vi "test2-DifferentChainNodesProcessDifferentAllowedMessages.vi"(8 "error in (no error)":errorcluster, 11 "TestCase in":refnum<class "testcase-CSMChainMode.lvclass">) -> (0 "error out":errorcluster, 3 "TestCase out":refnum<class "testcase-CSMChainMode.lvclass">)   [LabVIEW 2017, in "testcase-CSMChainMode.lvclass"]
uses:
  testcase-CSMChainMode.lvclass
  <vilib>/addons/_JKI Toolkits/VI Tester/TestCase.llb/TestCase.lvclass
  src/user.lib/_NEVSTOP/Communicable State Machine(CSM)/Communicable State Machine.lvlib
  C:/Program Files (x86)/National Instruments/LabVIEW 2017/vi.lib/addons/_JKI Toolkits/VI Tester/TestCase.llb/TestCase.lvclass
panel:
  out "LoopCount":i32
  out "error out 2":errorcluster
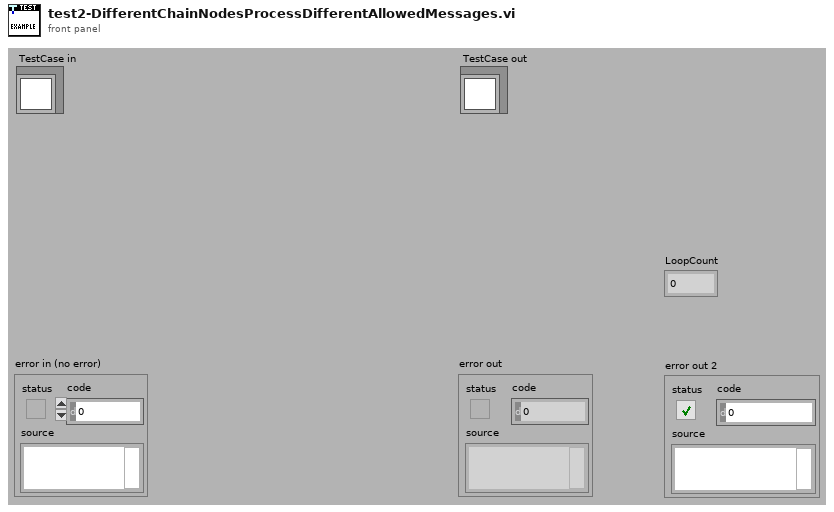
[diagram p1: front panel]
types:
  T1 = cluster{"Allowed":string, "Not Allowed":string[]}[]
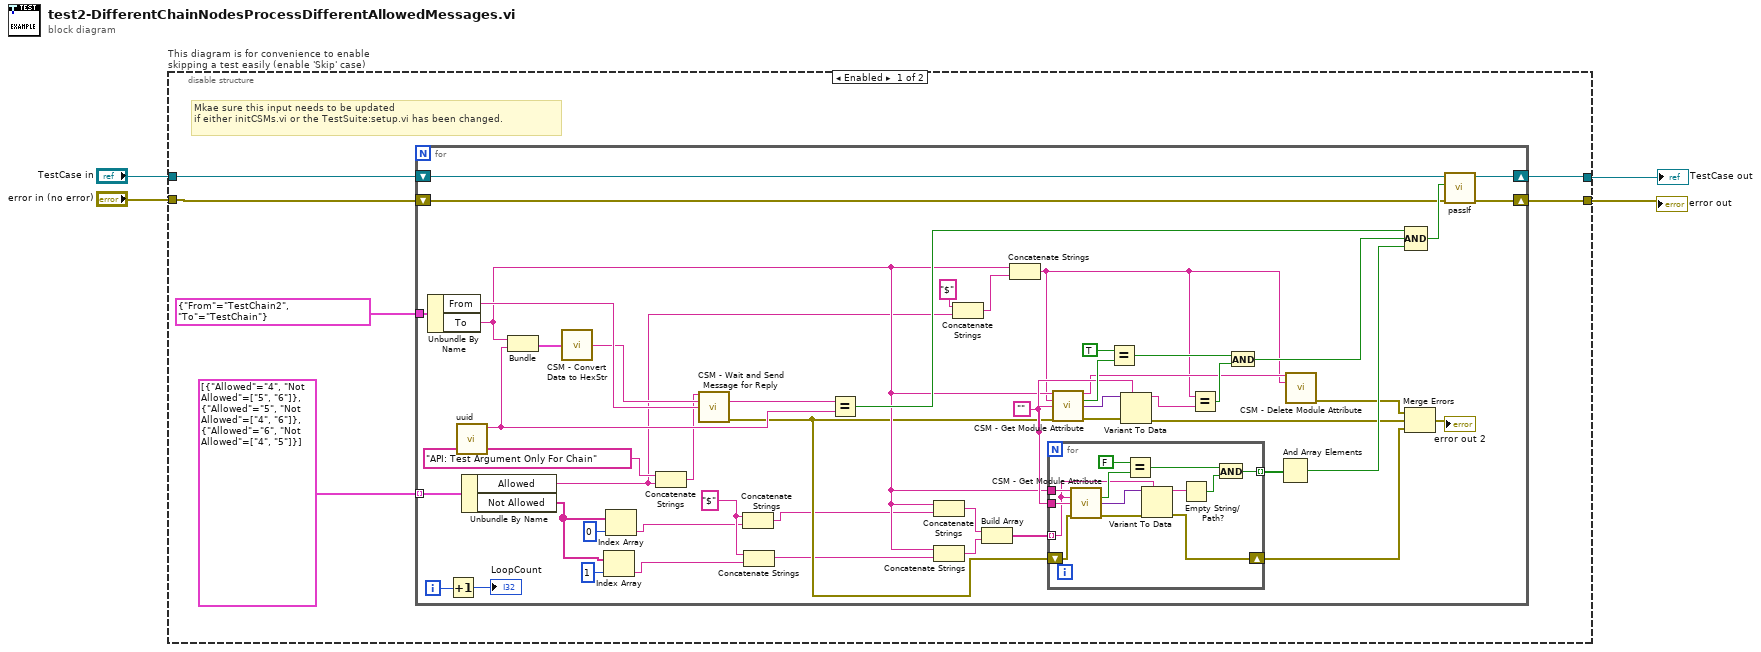
[diagram p0: block diagram]
diagram:
  n1 = disable-structure "This diagram is for convenience to enable skipping a test easily (enable 'Skip' case)" shown="Enabled" {
    disable-tunnel: "TestCase in" -> [w9 w77]
    disable-tunnel: [w7 w75] -> w1
    disable-tunnel: [w6 w76] -> w3
    disable-tunnel: "error in (no error)" -> [w8 w74]
    frame Enabled {
      # "Mkae sure this input needs to be updated \nif either initCSMs.vi or the TestSuite:setup.vi has been changed."
      n2 = for {
        tunnel: cluster{"From":string, "To":string} {"From"="TestChain2", "To"="TestChain"} ("Cluster") -> [w60]
        shift-right: [w52] -> w7
        shift-left: w9 -> [w56]
        shift-right: [w51] -> w6
        shift-left: w8 -> [w53]
        tunnel: T1 [{"Allowed"="4", "Not Allowed"=["5", "6"]}, {"Allowed"="5", "Not Allowed"=["4", "6"]}, {"Allowed"="6", "Not Allowed"=["4", "5"]}] -> [w27] mode=indexing
        i -> [w29]
        w21 = "$" ("string")
        w40 = ""
        n3 = Unbundle By Name(w60) -> ("From"=w59:string, "To"=w39:string)
        n4 = Increment(x=w29) -> (x+1=→"LoopCount":i32)
        n5 = call "uuid.vi"() -> ("UUID"=w43:string)  [unwired: 11 in]
        n6 = Unbundle By Name(w27) -> ("Allowed"=w23:string, "Not Allowed"=w17:string[])
        n7 = Bundle("To"=w39, "UUID"=w43) -> (w58:cluster{"To":string, "UUID":string})  [unwired: 1 in]
        n8 = call "CSM - Convert Data to HexStr.vi"("Variant"=w58) -> ("HEX String (0-9,A-F)"=w57:string)  [unwired: 8 in]
        n9 = Index Array(array=w17, index=1) -> (element=w16:string)
        n10 = Index Array(array=w17, index=0) -> (element=w19:string)
        n11 = Concatenate Strings("API: Test Argument Only For Chain" ("State"), w23) -> (w25:string)
        n12 = call "CSM - Wait and Send Message for Reply.vi"("State"=w25, "Arguments (\"\")"=w57, "Target Module"=w59) -> ("Response"=w44:string, "error out"=w33:errorcluster)  [unwired: 9 in, 2 out]
        n13 = Concatenate Strings(w21, w19) -> (w15:string)
        n14 = Concatenate Strings(w21, w16) -> (w14:string)
        n15 = Equal?(x=w44, y=w43) -> (x = y?=w55:bool)
        n16 = Concatenate Strings(w39, w15) -> (w38:string)
        n17 = Concatenate Strings(w39, w14) -> (w37:string)
        n18 = Concatenate Strings("$" ("string"), w23) -> (w22:string)
        n19 = Build Array(w38, w37) -> (w36:string[])
        n20 = Concatenate Strings(w39, w22) -> (w12:string)
        n21 = for {
          tunnel: w40 -> [w73]
          tunnel: w39 -> [w68]
          tunnel: w36 -> [w67] mode=indexing
          tunnel: [w63] -> w35 mode=indexing
          shift-right: [w61] -> w31
          shift-left: w33 -> [w62]
          n22 = call "CSM - Get Module Attribute.vi"("CSM Name"=w68, "Attribute"=w67, "Default Value (Empty Variant)"=w73, "Error In"=w62) -> ("Found"=w70:bool, "Value"=w71:variant, "error out"=w72:errorcluster)  [unwired: 7 in, 2 out]
          n23 = Equal?(x=FALSE, y=w70) -> (x = y?=w64:bool)
          n24 = Variant To Data(error in=w72, type=w67, Variant=w71) -> (data=w66:string, error out=w61:errorcluster)
          n25 = Empty String/Path?(string/path=w66) -> (empty?=w65:bool)
          n26 = And(x=w64, y=w65) -> (x .and. y?=w63:bool)
        }
        n27 = call "CSM - Get Module Attribute.vi"("CSM Name"=w39, "Attribute"=w12, "Default Value (Empty Variant)"=w40, "Error In"=w33) -> ("CSM Name (Dup)"=w13:string, "Found"=w50:bool, "Value"=w47:variant, "error out"=w48:errorcluster)  [unwired: 7 in, 1 out]
        n28 = Equal?(x=TRUE, y=w50) -> (x = y?=w46:bool)
        n29 = Variant To Data(error in=w48, type=w40, Variant=w47) -> (data=w42:string, error out=w32:errorcluster)
        n30 = Equal?(x=w12, y=w42) -> (x = y?=w45:bool)
        n31 = And(x=w46, y=w45) -> (x .and. y?=w41:bool)
        n32 = And Array Elements(Boolean array=w35) -> (logical AND=w34:bool)
        n33 = call "CSM - Delete Module Attribute.vi"("CSM Name"=w13, "Attribute"=w12) -> ("error out"=w11:errorcluster)  [unwired: 10 in, 3 out]
        n34 = Compound Arithmetic op=AND(w55, w41, w34) -> (w54:bool)
        n35 = Merge Errors(w11, w32, w31) -> (→"error out 2":errorcluster)
        n36 = call-dynamic "passIf.vi"("error in (no error)"=w53, "pass"=w54, "TestCase in"=w56) -> ("error out"=w51:errorcluster, "TestCase out"=w52:refnum<class "testcase-CSMChainMode.lvclass">)  [unwired: 7 in]
      }
    }
    frame Disabled {
      # "skip test result while test is under development"
      n37 = call <vilib>:"skip.vi"("error in (no error)"=w74, "TestCase in"=w77) -> ("error out"=w76:errorcluster, "TestCase out"=w75:refnum<class "testcase-CSMChainMode.lvclass">)  [unwired: 8 in]
    }
  }
  "error out" <- w3
  "TestCase out" <- w1
